vi "InitiateNotifiers.vi"(2 "error in (no error)":errorcluster, 3 "Boat Type":T1(ring)) -> (0 "error out":errorcluster, 1 "NotifierReferences":T2)   [LabVIEW 2013]
doc: "Initializes all the notifiers that will be used to pass data around."
uses:
  Data/TypeDefs/Notifiers.ctl
  Data/TypeDefs/UTM Location.ctl
  Data/TypeDefs/GPS Sensor Status.ctl
  Data/TypeDefs/Sail Set Suggestions.ctl
  Data/TypeDefs/Rudder Set Suggestions.ctl
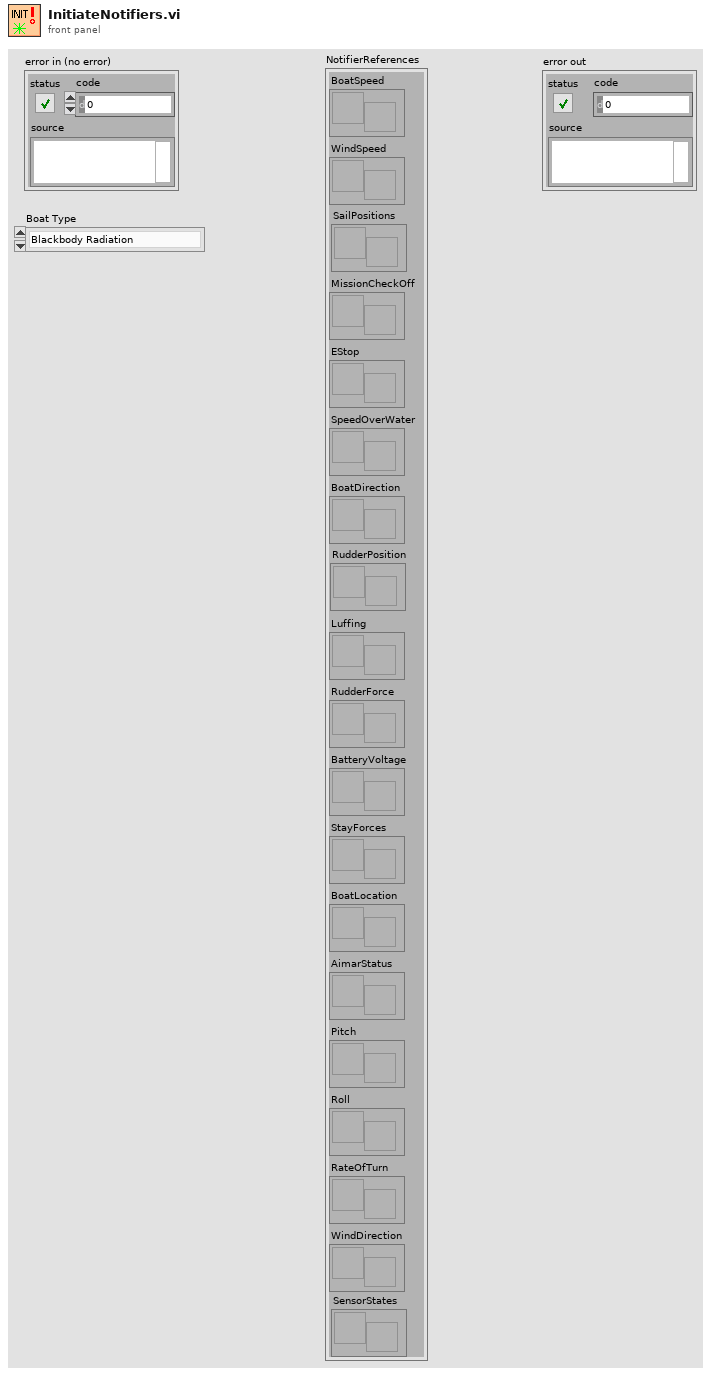
[diagram p1: front panel]
types:
  T1 = enum16{"Blackbody Radiation", "Little boats", "Simulation", "Damn Yankee"}
  T2 = typedef "Notifiers.ctl" = cluster{"BoatSpeed":refnum<notifier>, "WindSpeed":refnum<notifier>, "MissionCheckOff":refnum<notifier>, "EStop":refnum<notifier>, "SpeedOverWater":refnum<notifier>, "BoatDirection":refnum<notifier>, "Luffing":refnum<notifier>, "RudderForce":refnum<notifier>, "BatteryVoltage":refnum<notifier>, "StayForces":refnum<notifier>, "BoatLocation":refnum<notifier>, "AimarStatus":refnum<notifier>, "Pitch":refnum<notifier>, "Roll":refnum<notifier>, "RateOfTurn":refnum<notifier>, "WindDirection":refnum<notifier>, "SailPositions":refnum<notifier>, "RudderPosition":refnum<notifier>, "SensorStates":refnum<notifier>}
  T3 = cluster{"AirmarOnline":bool, "WindvaneOnline":bool, "HemisphereOnline":bool, "RudderForceOnline":bool, "StayForceOnline":bool, "BatteryVoltageOnline":bool, "AccelerometerOnline":bool}
  T4 = typedef "Rudder Set Suggestions.ctl" = dbl
  T5 = typedef "Sail Set Suggestions.ctl" = cluster{"MainSailSuggestion":dbl, "JibSailSuggestion":dbl}
  T6 = typedef "GPS Sensor Status.ctl" = cluster{"Sensor Connected":bool, "Sensor OK":bool, "GPS Lock":bool, "Sensor Initialized":bool}
  T7 = typedef "UTM Location.ctl" = cluster{"UTM Zone":dbl, "Hemisphere":enum16{"North", "South"}, "East":dbl, "North":dbl}
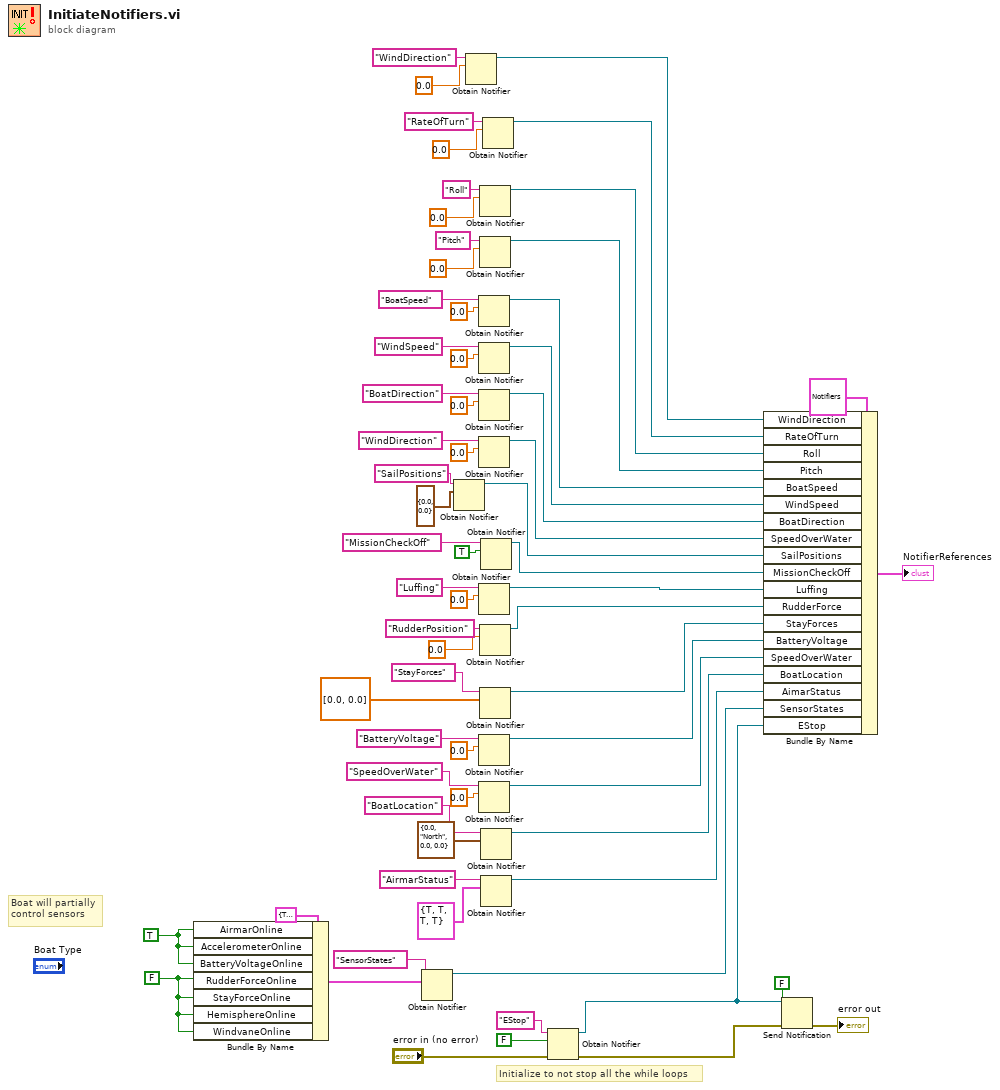
[diagram p0: block diagram]
diagram:
  w4 = FALSE ("AirmarOnline")
  w5 = TRUE ("AirmarOnline")
  # "Boat will partially\ncontrol sensors"
  # "Initialize to not stop all the while loops"
  n1 = Bundle By Name(cluster=T3 {"AirmarOnline"=TRUE, "WindvaneOnline"=TRUE, "HemisphereOnline"=TRUE, "RudderForceOnline"=TRUE, "StayForceOnline"=TRUE, "BatteryVoltageOnline"=TRUE, "AccelerometerOnline"=TRUE}, "AirmarOnline"=w5, "AccelerometerOnline"=w5, "BatteryVoltageOnline"=w5, "RudderForceOnline"=w4, "StayForceOnline"=w4, "HemisphereOnline"=w4, "WindvaneOnline"=w4) -> (w3:T3)
  n2 = Obtain Notifier(name (unnamed)="SensorStates", notification data type=w3) -> (notifier out=w1:refnum<notifier>)  [unwired: 2 in, 2 out]
  n3 = Obtain Notifier(name (unnamed)="SailPositions", notification data type=T5 {"MainSailSuggestion"=0.0, "JibSailSuggestion"=0.0} ("output cluster")) -> (notifier out=w9:refnum<notifier>)  [unwired: 2 in, 2 out]
  n4 = Obtain Notifier(name (unnamed)="WindDirection", notification data type=0.0) -> (notifier out=w14:refnum<notifier>)  [unwired: 2 in, 2 out]
  n5 = Obtain Notifier(name (unnamed)="BoatSpeed", notification data type=0.0) -> (notifier out=w58:refnum<notifier>)  [unwired: 2 in, 2 out]
  n6 = Obtain Notifier(name (unnamed)="WindSpeed", notification data type=0.0) -> (notifier out=w57:refnum<notifier>)  [unwired: 2 in, 2 out]
  n7 = Obtain Notifier(name (unnamed)="BoatDirection", notification data type=0.0) -> (notifier out=w56:refnum<notifier>)  [unwired: 2 in, 2 out]
  n8 = Obtain Notifier(name (unnamed)="WindDirection", notification data type=0.0) -> (notifier out=w55:refnum<notifier>)  [unwired: 2 in, 2 out]
  n9 = Obtain Notifier(name (unnamed)="Luffing", notification data type=0.0) -> (notifier out=w39:refnum<notifier>)  [unwired: 2 in, 2 out]
  n10 = Obtain Notifier(name (unnamed)="BatteryVoltage", notification data type=0.0) -> (notifier out=w36:refnum<notifier>)  [unwired: 2 in, 2 out]
  n11 = Obtain Notifier(name (unnamed)="SpeedOverWater", notification data type=0.0) -> (notifier out=w35:refnum<notifier>)  [unwired: 2 in, 2 out]
  n12 = Obtain Notifier(name (unnamed)="Roll", notification data type=0.0) -> (notifier out=w20:refnum<notifier>)  [unwired: 2 in, 2 out]
  n13 = Obtain Notifier(name (unnamed)="Pitch", notification data type=0.0) -> (notifier out=w23:refnum<notifier>)  [unwired: 2 in, 2 out]
  n14 = Obtain Notifier(name (unnamed)="RudderPosition", notification data type=T4 0.0 ("Suggested Rudder Setpoint")) -> (notifier out=w8:refnum<notifier>)  [unwired: 2 in, 2 out]
  n15 = Obtain Notifier(name (unnamed)="StayForces", notification data type=dbl[] [0.0, 0.0] ("Array")) -> (notifier out=w37:refnum<notifier>)  [unwired: 2 in, 2 out]
  n16 = Obtain Notifier(name (unnamed)="MissionCheckOff", notification data type=TRUE) -> (notifier out=w54:refnum<notifier>)  [unwired: 2 in, 2 out]
  n17 = Obtain Notifier(name (unnamed)="BoatLocation", notification data type=T7 {"UTM Zone"=0.0, "Hemisphere"=enum."North", "East"=0.0, "North"=0.0} ("UTM Location")) -> (notifier out=w29:refnum<notifier>)  [unwired: 2 in, 2 out]
  n18 = Obtain Notifier(name (unnamed)="AirmarStatus", notification data type=T6 {"Sensor Connected"=TRUE, "Sensor OK"=TRUE, "GPS Lock"=TRUE, "Sensor Initialized"=TRUE} ("input cluster")) -> (notifier out=w26:refnum<notifier>)  [unwired: 2 in, 2 out]
  n19 = Obtain Notifier(name (unnamed)="RateOfTurn", notification data type=0.0) -> (notifier out=w17:refnum<notifier>)  [unwired: 2 in, 2 out]
  n20 = Obtain Notifier(name (unnamed)="EStop", notification data type=FALSE, error in (no error)="error in (no error)") -> (notifier out=w2:refnum<notifier>, error out=w51:errorcluster)  [unwired: 1 in, 1 out]
  n21 = Bundle By Name(cluster=T2 {"BoatSpeed"=refnum, "WindSpeed"=refnum, "MissionCheckOff"=refnum, "EStop"=refnum, "SpeedOverWater"=refnum, "BoatDirection"=refnum, "Luffing"=refnum, "RudderForce"=refnum, "BatteryVoltage"=refnum, "StayForces"=refnum, "BoatLocation"=refnum, "AimarStatus"=refnum, "Pitch"=refnum, "Roll"=refnum, "RateOfTurn"=refnum, "WindDirection"=refnum, "SailPositions"=refnum, "RudderPosition"=refnum, "SensorStates"=refnum} ("NotifierReff 2"), "WindDirection"=w14, "RateOfTurn"=w17, "Roll"=w20, "Pitch"=w23, "BoatSpeed"=w58, "WindSpeed"=w57, "BoatDirection"=w56, "SpeedOverWater"=w55, "SailPositions"=w9, "MissionCheckOff"=w54, "Luffing"=w39, "RudderForce"=w8, "StayForces"=w37, "BatteryVoltage"=w36, "SpeedOverWater"=w35, "BoatLocation"=w29, "AimarStatus"=w26, "SensorStates"=w1, "EStop"=w2) -> (→"NotifierReferences":T2)
  n22 = Send Notification(notification=FALSE, notifier=w2, error in (no error)=w51) -> (error out=→"error out":errorcluster)  [unwired: 1 out]
